vi "DB_EscribeTablaUsuarios.vi"(0 "NOMBRE":string, 1 "APELLIDO":string, 2 "USUARIO":string, 3 "PASS":string, 4 "CATEGORIA":string(combo), 5 "error in (no error)":errorcluster) -> (14 "FECHA REGISTRO":string, 19 "error out":errorcluster)   [LabVIEW 2018]
uses:
  <vilib>/addons/database/Connection.llb/DB Tools Open Connec (Path).vi
  <vilib>/addons/database/Connection.llb/Conn Execute.vi
  <vilib>/addons/database/Recordset.llb/Rec Destroy - Connection.vi
  <vilib>/addons/database/NI_Database_API.lvlib
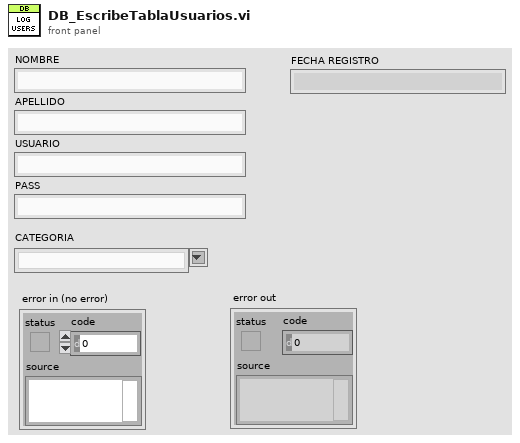
[diagram p1: front panel]
types:
  T1 = typedef "NI_Database_API.lvlib/Conn ObjectReference.ctl" = refnum<k1>
  T2 = typedef "NI_Database_API.lvlib/Rec ObjectReference.ctl" = refnum<k1>
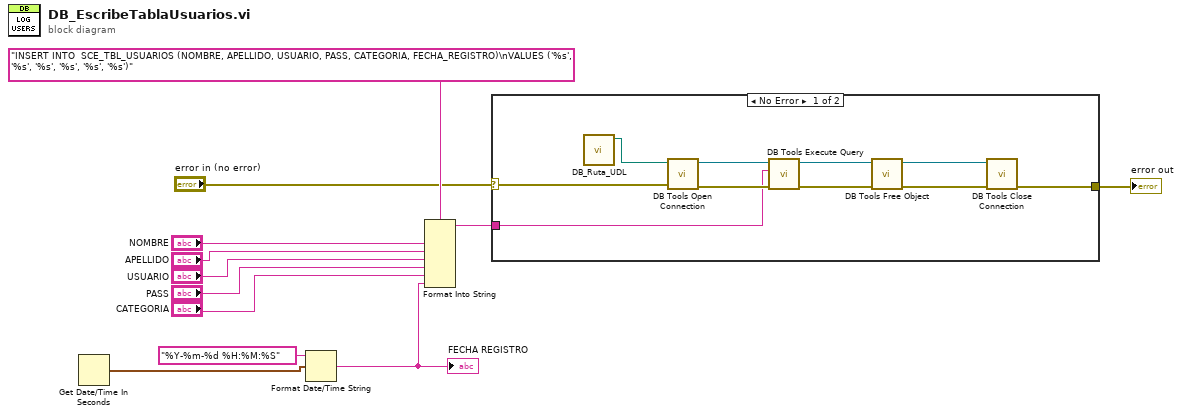
[diagram p0: block diagram]
diagram:
  n1 = Get Date/Time In Seconds() -> (seconds since 1Jan1904=w3:timestamp)
  n2 = Format Date/Time String(time format string (%c)="%Y-%m-%d %H:%M:%S", seconds (now)=w3) -> (date/time string=w2:string)  [unwired: 1 in]
  "FECHA REGISTRO" <- w2
  n3 = Format Into String(format string="INSERT INTO  SCE_TBL_USUARIOS (NOMBRE, APELLIDO, USUARIO, PASS, CATEGORIA, FECHA_REGISTRO)\nVALUES ('%s', '%s', '%s', '%s', '%s', '%s')" ("SQL"), "NOMBRE", "APELLIDO", "USUARIO", "PASS", "CATEGORIA", w2) -> (resulting string=w12:string)  [unwired: 2 in, 1 out]
  n4 = case shown="No Error" "error in (no error)" {
    selector: "error in (no error)" -> [w15 w23]
    tunnel: w12 -> [w19 _]
    tunnel: [w16 w23] -> w10
    frame No Error {
      n5 = call "DB_Ruta_UDL.vi"() -> ("UDL ruta"=w14:path)  [unwired: 11 in]
      n6 = call-poly <vilib>:"DB Tools Open Connection.vi"("error in (no error)"=w15, "connection information"=w14) -> ("error out"=w22:errorcluster, "connection reference"=w20:T1)  [unwired: 6 in]
      n7 = call-poly <vilib>:"DB Tools Execute Query.vi"("error in (no error)"=w22, "SQL query"=w19, "connection reference"=w20) -> ("error out"=w21:errorcluster, "recordset reference"=w17:T2)  [unwired: 5 in]
      n8 = call-poly <vilib>:"DB Tools Free Object.vi"("error in (no error)"=w21, "recordset reference"=w17) -> ("error out"=w18:errorcluster, "connection reference"=w13:T1)  [unwired: 8 in]
      n9 = call <vilib>:"DB Tools Close Connection.vi"("error in (no error)"=w18, "connection reference"=w13) -> ("error out"=w16:errorcluster)  [unwired: 5 in]
    }
    frame Error {
    }
  }
  "error out" <- w10
